vi "Write Data OK_.vi"(8 "error in (no error)":errorcluster, 10 "Data OK?":bool, 11 "Instrument in":refnum<class "Instrument.lvclass">) -> (0 "error out":errorcluster, 3 "Instrument out":refnum<class "Instrument.lvclass">)   [LabVIEW 2014, in "Instrument.lvclass"]
uses:
  Instrument.lvclass
  Instrument.lvclass/Instrument.ctl
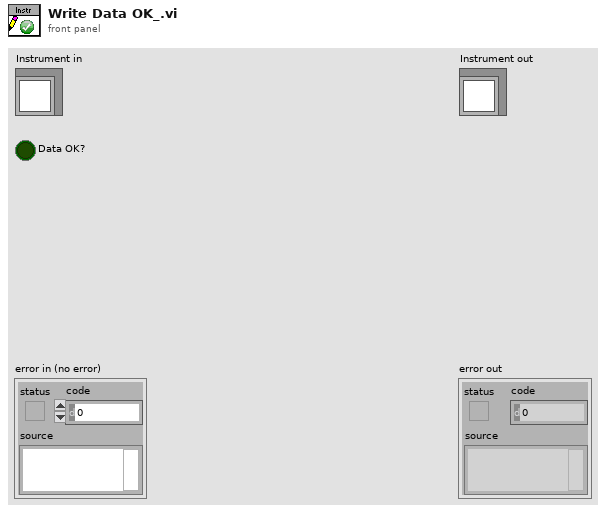
[diagram p1: front panel]
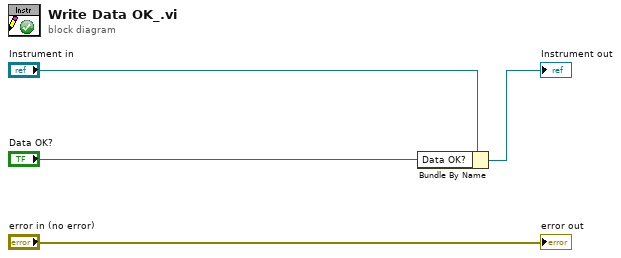
[diagram p0: block diagram]
diagram:
  n1 = Bundle By Name(cluster="Instrument in", "Data OK?"="Data OK?") -> (→"Instrument out":refnum<class "Instrument.lvclass">)
  "error out" <- "error in (no error)"
